vi "picoToVolts.vi"(8 "error in (no error)":errorcluster, 9 "Max_adc":i16=32767, 10 "Range Index":u16, 11 "Data":dbl[](array[numeric])) -> (0 "error out":errorcluster, 3 "Data (mV)":dbl[](array[numeric]))   [LabVIEW 2011]
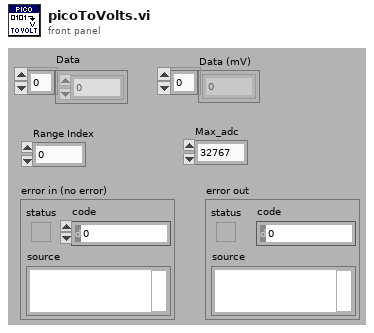
[diagram p1: front panel]
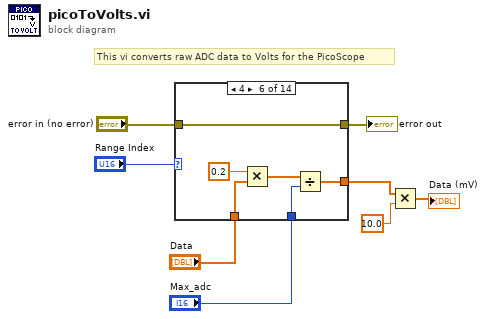
[diagram p0: block diagram]
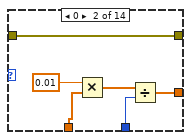
[diagram p3: hidden frame]
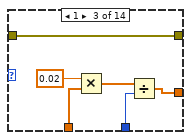
[diagram p4: hidden frame]
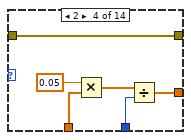
[diagram p5: hidden frame]
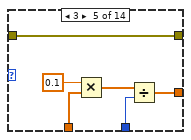
[diagram p6: hidden frame]
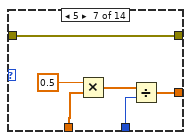
[diagram p7: hidden frame]
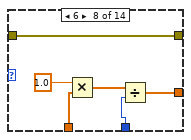
[diagram p8: hidden frame]
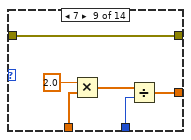
[diagram p9: hidden frame]
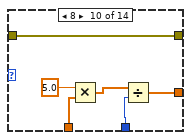
[diagram p10: hidden frame]
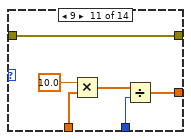
[diagram p11: hidden frame]
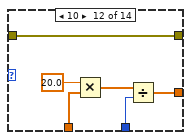
[diagram p12: hidden frame]
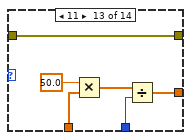
[diagram p13: hidden frame]
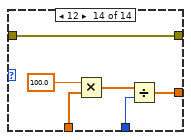
[diagram p14: hidden frame]
diagram:
  # "This vi converts raw ADC data to Volts for the PicoScope"
  n1 = case shown="4" "Range Index" {
    tunnel: [w10 w14 w19 w26 w32 w38 w44 w49 w56 w62 w68 w74 w80 w86] -> w3
    tunnel: "Data" -> [w10 w12 w20 w25 w31 w37 w43 w50 w55 w61 w67 w73 w79 w85]
    tunnel: "Max_adc" -> [_ w13 w18 w24 w30 w36 w42 w48 w54 w60 w66 w72 w78 w84]
    tunnel: "error in (no error)" -> [w9 w11 w17 w23 w29 w35 w41 w47 w53 w59 w65 w71 w77 w83]
    tunnel: [w9 w11 w17 w23 w29 w35 w41 w47 w53 w59 w65 w71 w77 w83] -> w4
    frame Default {
    }
    frame 0 {
      n2 = Multiply(x=0.01, y=w12) -> (x*y=w15:dbl[])
      n3 = Divide(x=w15, y=w13) -> (x/y=w14:dbl[])
    }
    frame 1 {
      n4 = Multiply(x=0.02, y=w20) -> (x*y=w22:dbl[])
      n5 = Divide(x=w22, y=w18) -> (x/y=w19:dbl[])
    }
    frame 2 {
      n6 = Multiply(x=0.05, y=w25) -> (x*y=w27:dbl[])
      n7 = Divide(x=w27, y=w24) -> (x/y=w26:dbl[])
    }
    frame 3 {
      n8 = Multiply(x=0.1, y=w31) -> (x*y=w33:dbl[])
      n9 = Divide(x=w33, y=w30) -> (x/y=w32:dbl[])
    }
    frame 4 {
      n10 = Multiply(x=0.2, y=w37) -> (x*y=w40:dbl[])
      n11 = Divide(x=w40, y=w36) -> (x/y=w38:dbl[])
    }
    frame 5 {
      n12 = Multiply(x=0.5, y=w43) -> (x*y=w46:dbl[])
      n13 = Divide(x=w46, y=w42) -> (x/y=w44:dbl[])
    }
    frame 6 {
      n14 = Multiply(x=1.0, y=w50) -> (x*y=w52:dbl[])
      n15 = Divide(x=w52, y=w48) -> (x/y=w49:dbl[])
    }
    frame 7 {
      n16 = Multiply(x=2.0, y=w55) -> (x*y=w58:dbl[])
      n17 = Divide(x=w58, y=w54) -> (x/y=w56:dbl[])
    }
    frame 8 {
      n18 = Multiply(x=5.0, y=w61) -> (x*y=w64:dbl[])
      n19 = Divide(x=w64, y=w60) -> (x/y=w62:dbl[])
    }
    frame 9 {
      n20 = Multiply(x=10.0, y=w67) -> (x*y=w70:dbl[])
      n21 = Divide(x=w70, y=w66) -> (x/y=w68:dbl[])
    }
    frame 10 {
      n22 = Multiply(x=20.0, y=w73) -> (x*y=w76:dbl[])
      n23 = Divide(x=w76, y=w72) -> (x/y=w74:dbl[])
    }
    frame 11 {
      n24 = Multiply(x=50.0, y=w79) -> (x*y=w82:dbl[])
      n25 = Divide(x=w82, y=w78) -> (x/y=w80:dbl[])
    }
    frame 12 {
      n26 = Multiply(x=100.0, y=w85) -> (x*y=w88:dbl[])
      n27 = Divide(x=w88, y=w84) -> (x/y=w86:dbl[])
    }
  }
  "error out" <- w4
  n28 = Multiply(x=w3, y=10.0 ("x")) -> (x*y=→"Data (mV)":dbl[])
